vi "Cleanup.vi"(8 "error in (no error)":errorcluster, 11 "MuxPanel in":refnum<class "MuxPanel.lvclass">) -> (0 "error out":errorcluster)   [LabVIEW 2022 SP3, in "TouchControl.lvlib" / "MuxPanel.lvclass"]
uses:
  MuxPanel.lvclass
  MuxPanel.lvclass/MuxPanel.ctl
  <vilib>/IlluminatedG/IG OOPanel/OOPanel/Panel/Panel.lvclass
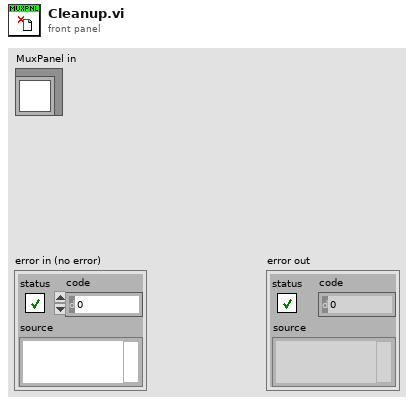
[diagram p1: front panel]
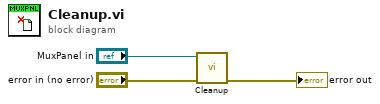
[diagram p0: block diagram]
diagram:
  n1 = call-parent "Cleanup.vi"("error in (no error)"="error in (no error)", "Panel in"="MuxPanel in") -> ("error out"=→"error out":errorcluster)  [unwired: 9 in]
